vi "Forebrain.vi"() -> ()   [LabVIEW 2012]
uses:
  <vilib>/Utility/inputDevices.llb/closeKeyboard.vi
  <vilib>/Utility/inputDevices.llb/keyboardAcquire.vi
panel:
  in  "MANUAL \nOVERRIDE":bool
  out "Starboard Speed":i32(knob) scale=1000.0..2000.0
  out "Port Speed":i32(knob) scale=1000.0..2000.0
  in  "Rudders":i32(slide)=1500 scale=500.0..2500.0
  in  "Step Size":i32=5
  out "Speed                    Balance":i32(knob) scale=-1000.0..1000.0
  in  "Pan Camera":i32(slide)=1500 scale=500.0..2500.0
  in  "FULL STOP":bool
  out "UDP Timeout":bool
  out "UDP Working":bool
  in  "ESTOP":bool
  in  "PC Status":i32=1
  out "Port Rudder":i32
  out "Starboard Rudder":i32
  out "Port Motor":i32
  out "Starboard Motor":i32
  out "Data from XBEE":dbl
  out "XBEE Working":bool
  out "return count":u32
  out "Sent from XBEE":string
  out "bytes written":u32
  in  "Send to XBEE":string
  in  "VISA resource name":refnum<visa-resource-name>="COM6"
  in  "error in":errorcluster
  out "Base Station data rec'd":string
  out "Robot Stats":i32[](array[numeric])
  out "Buoy locations":cluster{"regular expression":string, i32, i32}[](array[cluster])
  # "ORGANIZE FRONT PANEL"
  # "Tug X"
  # "Tug Y"
  # "Tug H"
  # "MANUAL OVERRIDE CONTROLS"
  # "Controls:\nUse W/S to independently\ncontrol port speed.\nUse I/K to independently\ncontrol starboard speed.\nUse arrow keys to jointly\ncontrol motor speeds.\n\nUSE ESCAPE TO KILL MOTORS."
  # "Affects weight of single key input."
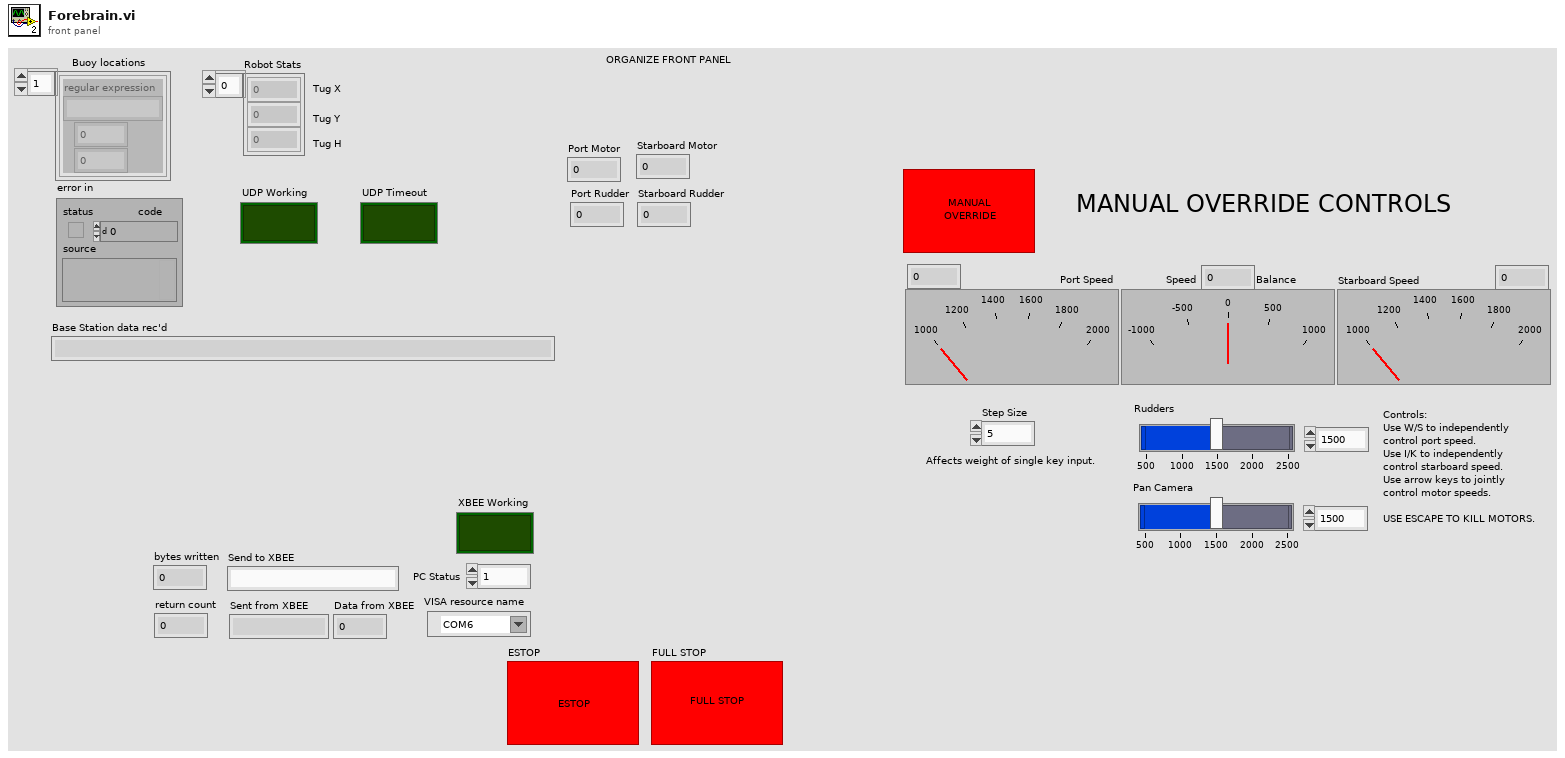
[diagram p1: front panel]
types:
  T1 = enum16{"0", "1", "2", "3", "4", "5", "6", "7", "8", "9", "A", "B", "C", "D", "E", "F", "G", "H", "I", "J", "K", "L", "M", "N", "O", "P", "Q", "R", "S", "T", "U", "V", "W", "X", "Y", "Z", "F1", "F2", "F3", "F4", "F5", "F6", "F7", "F8", "F9", "F10", "F11", "F12", "F13", "F14", "F15", "ADD", "BACK", "BACKSLASH", "CAPITAL", "COMMA", "DECIMAL", "DELETE", "DIVIDE", "DOWN", "END", "EQUALS", "ESCAPE", "GRAVE (`)", "HOME", "INSERT", "LBRACKET", "LCONTROL", "LEFT", "L ALT", "LSHIFT", "LWIN", "MINUS", "MULTIPLY", "NEXT", "NUMLOCK", "NUMPAD_0", "NUMPAD_1", "NUMPAD_2", "NUMPAD_3", "NUMPAD_4", "NUMPAD_5", "NUMPAD_6", "NUMPAD_7", "NUMPAD_8", "NUMPAD_9", "PAUSE", "PERIOD", "PRIOR (PG UP)", "RBRACKET", "RCONTROL", "RETURN", "RIGHT", "R ALT", "RSHIFT", "RWIN", "SCROLL", "SEMICOLON", "SLASH", "SPACE", "SUBTRACT", "TAB", "UP", "ENTER (num pad)", "' (quote)"}[]
  T2 = enum16{"0", "1", "2", "3", "4", "5", "6", "7", "8", "9", "A", "B", "C", "D", "E", "F", "G", "H", "I", "J", "K", "L", "M", "N", "O", "P", "Q", "R", "S", "T", "U", "V", "W", "X", "Y", "Z", "F1", "F2", "F3", "F4", "F5", "F6", "F7", "F8", "F9", "F10", "F11", "F12", "F13", "F14", "F15", "ADD", "BACK", "BACKSLASH", "CAPITAL", "COMMA", "DECIMAL", "DELETE", "DIVIDE", "DOWN", "END", "EQUALS", "ESCAPE", "GRAVE (`)", "HOME", "INSERT", "LBRACKET", "LCONTROL", "LEFT", "L ALT", "LSHIFT", "LWIN", "MINUS", "MULTIPLY", "NEXT", "NUMLOCK", "NUMPAD_0", "NUMPAD_1", "NUMPAD_2", "NUMPAD_3", "NUMPAD_4", "NUMPAD_5", "NUMPAD_6", "NUMPAD_7", "NUMPAD_8", "NUMPAD_9", "PAUSE", "PERIOD", "PRIOR (PG UP)", "RBRACKET", "RCONTROL", "RETURN", "RIGHT", "R ALT", "RSHIFT", "RWIN", "SCROLL", "SEMICOLON", "SLASH", "SPACE", "SUBTRACT", "TAB", "UP", "ENTER (num pad)", "' (quote)"}
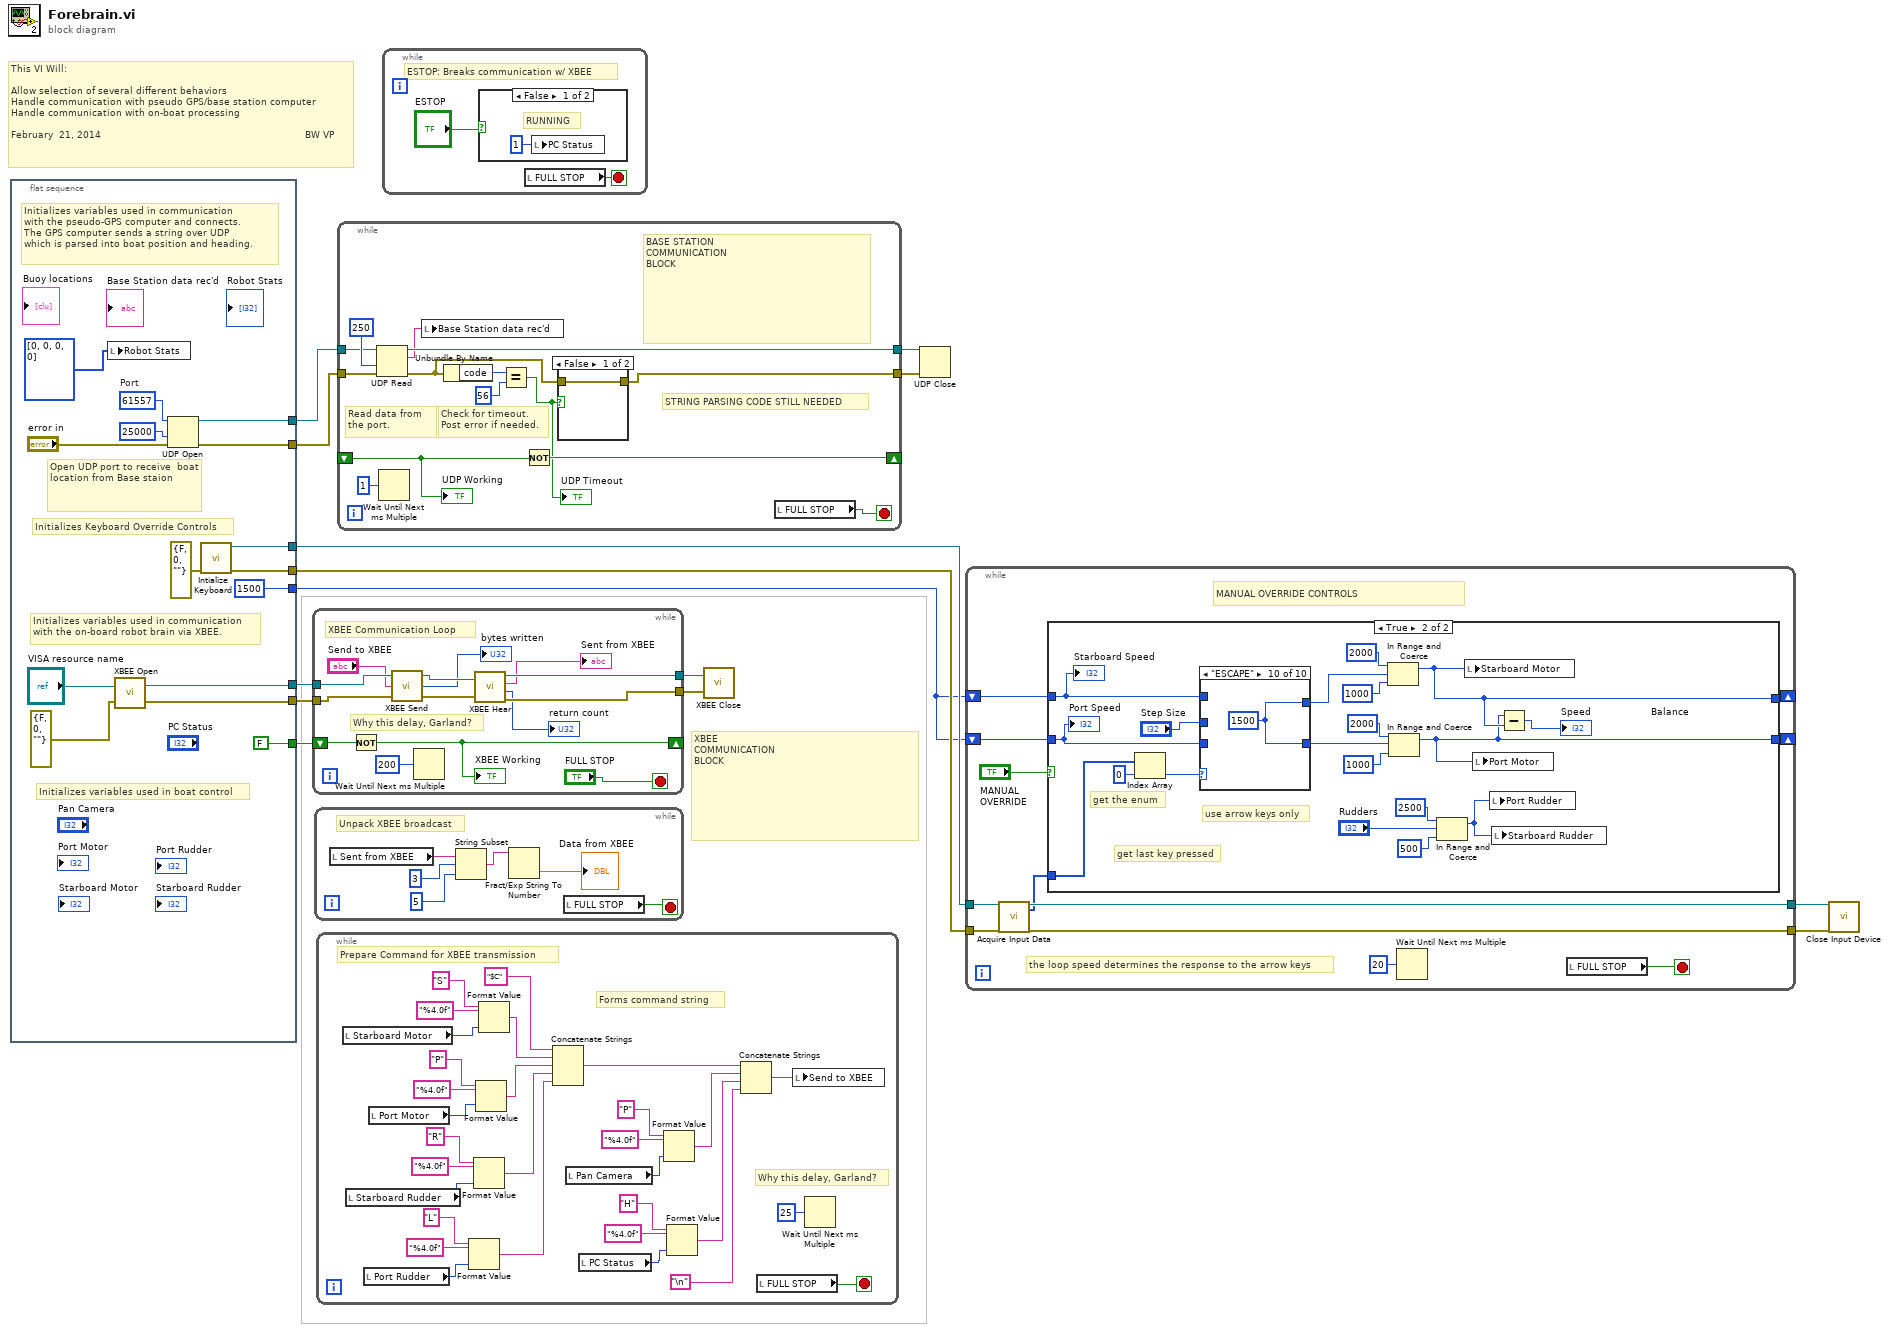
[diagram p0: block diagram]
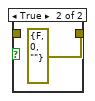
[diagram p2: hidden frame]
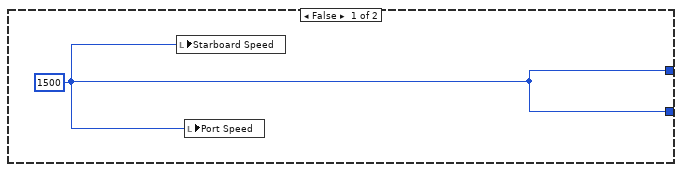
[diagram p3: hidden frame]
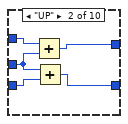
[diagram p5: hidden frame]
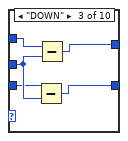
[diagram p6: hidden frame]
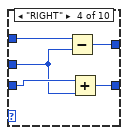
[diagram p7: hidden frame]
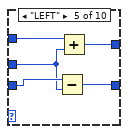
[diagram p8: hidden frame]
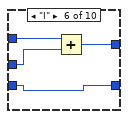
[diagram p9: hidden frame]
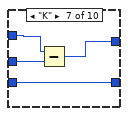
[diagram p10: hidden frame]
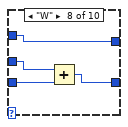
[diagram p11: hidden frame]
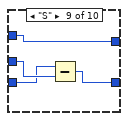
[diagram p12: hidden frame]
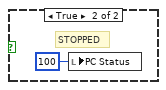
[diagram p13: hidden frame]
diagram:
  # "XBEE \nCOMMUNICATION\nBLOCK"
  # "This VI Will:\n\nAllow selection of several different behaviors\nHandle communication with pseudo GPS/base station computer\nHandle communication with on-boat processing\n\nFebruary  21, 2014                                                                    BW VP"
  n1 = flat-sequence {
    tunnel: [w25] -> w2
    tunnel: [w24] -> w1
    tunnel: [w21] -> w14
    tunnel: [w20] -> w13
    tunnel: [FALSE] -> w10
    tunnel: [w17] -> w7
    tunnel: [w16] -> w6
    tunnel: [1500] -> w5
    frame #0 {
      w28 = u16 61557  # Port
      # "Initializes Keyboard Override Controls"
      # "Initializes variables used in boat control"
      # "Initializes variables used in communication\nwith the on-board robot brain via XBEE."
      # "Initializes variables used in communication\nwith the pseudo-GPS computer and connects.\nThe GPS computer sends a string over UDP\nwhich is parsed into boat position and heading."
      # "Open UDP port to receive  boat location from Base staion"
      n2 = local write "Robot Stats"(i32[] [0, 0, 0, 0]) -> ()
      n3 = call "XBEE Open.vi"("error in"=errorcluster {"status"=FALSE, "code"=0, "source"=""}, "VISA resource name"="VISA resource name") -> ("error out"=w20:errorcluster, "VISA resource name out"=w21:refnum<visa-resource-name>)
      n4 = UDP Open(8:"error in", 9:25000 ("timeout ms (25000)"), 11:w28) -> (port=w25:refnum<k16>, 0:w24:errorcluster)  [unwired: 2 in, 1 out]
      n5 = call <vilib>:"Intialize Keyboard.vi"("error in (no error)"=errorcluster {"status"=FALSE, "code"=0, "source"=""}) -> ("error out"=w16:errorcluster, "device ID"=w17:refnum<k1>)  [unwired: 9 in]
    }
  }
  n6 = while {
    tunnel: w14 -> [w43]
    tunnel: w13 -> [w42]
    tunnel: [w37] -> w12
    tunnel: [w36] -> w11
    shift-right: [w31] -> _
    shift-left: w10 -> [w33]
    stop <- "FULL STOP" stop-if-true
    # "Why this delay, Garland?"
    # "XBEE Communication Loop"
    n7 = Not(x=w33) -> (.not. x?=w31:bool)
    "XBEE Working" <- w31
    n8 = call "XBEE Send.vi"("error in (no error)"=w42, "String"="Send to XBEE", "VISA resource name"=w43) -> ("error out"=w39:errorcluster, "return count"=→"bytes written":u32, "VISA resource name out"=w40:refnum<visa-resource-name>)
    n9 = Wait Until Next ms Multiple(millisecond multiple=200) -> ()  [unwired: 1 out]
    n10 = call "XBEE Hear.vi"("VISA resource name"=w40, "error in (no error)"=w39) -> ("VISA resource name out"=w37:refnum<visa-resource-name>, "String Received"=→"Sent from XBEE":string, "return count"=→"return count":u32, "error out"=w36:errorcluster)
  }
  n11 = while {
    stop <- w49 stop-if-true
    # "Unpack XBEE broadcast"
    n12 = local read "Sent from XBEE"() -> (w48:string)
    n13 = String Subset(string=w48, offset (0)=3, length (rest)=5 ("length (rest)")) -> (substring=w45:string)
    n14 = Fract/Exp String To Number(string=w45) -> (number=→"Data from XBEE":dbl)  [unwired: 3 in, 1 out]
    n15 = local read "FULL STOP"() -> (w49:bool)
  }
  n16 = while {
    stop <- w79 stop-if-true
    # "Why this delay, Garland?"
    # "Prepare Command for XBEE transmission"
    # "Forms command string"
    n17 = local read "Starboard Motor"() -> (w76:i32)
    n18 = local read "Starboard Rudder"() -> (w67:i32)
    n19 = local read "Port Rudder"() -> (w64:i32)
    n20 = local read "Port Motor"() -> (w73:i32)
    n21 = Format Value(string ("")="L", format string="%4.0f", value (0)=w64) -> (output string=w62:string)
    n22 = Format Value(string ("")="R", format string="%4.0f", value (0)=w67) -> (output string=w63:string)
    n23 = Format Value(string ("")="P", format string="%4.0f", value (0)=w73) -> (output string=w70:string)
    n24 = Format Value(string ("")="S", format string="%4.0f", value (0)=w76) -> (output string=w71:string)
    n25 = Concatenate Strings("$C", w71, w70, w63, w62) -> (w54:string)
    n26 = local read "Pan Camera"() -> (w58:i32)
    n27 = local read "PC Status"() -> (w55:i32)
    n28 = Format Value(string ("")="P", format string="%4.0f", value (0)=w58) -> (output string=w53:string)
    n29 = Format Value(string ("")="H", format string="%4.0f", value (0)=w55) -> (output string=w52:string)
    n30 = Concatenate Strings(w54, w53, w52, "\n") -> (w59:string)
    n31 = local read "FULL STOP"() -> (w79:bool)
    n32 = local write "Send to XBEE"(w59) -> ()
    n33 = Wait Until Next ms Multiple(millisecond multiple=u32 25) -> ()  [unwired: 1 out]
  }
  n34 = while {
    shift-right: [w91] -> _
    shift-left: _ -> [w81]
    tunnel: [w90] -> w4
    tunnel: [w86] -> w3
    tunnel: w2 -> [w84]
    tunnel: w1 -> [w83]
    stop <- w82 stop-if-true
    # "BASE STATION \nCOMMUNICATION\nBLOCK"
    # "Check for timeout.\nPost error if needed."
    # "Read data from\nthe port."
    # "STRING PARSING CODE STILL NEEDED"
    n35 = UDP Read(connection ID=w84, timeout ms (25000)=250, 8:w83) -> (data out=w85:string, error out=w87:errorcluster, 3:w90:refnum<k16>)  [unwired: 1 in, 2 out]
    n36 = Wait Until Next ms Multiple(millisecond multiple=u32 1) -> ()  [unwired: 1 out]
    n37 = local write "Base Station data rec'd"(w85) -> ()
    n38 = Unbundle By Name(w87) -> ("code"=w89:i32)
    n39 = Equal?(x=w89, y=56) -> (x = y?=w80:bool)
    "UDP Timeout" <- w80
    n40 = Not(x=w81) -> (.not. x?=w91:bool)
    n41 = case shown="False" w80 {
      tunnel: w87 -> [w94 _]
      tunnel: [w94 errorcluster {"status"=FALSE, "code"=0, "source"=""} ("error out")] -> w86
      frame False {
      }
      frame True {
      }
    }
    n42 = local read "FULL STOP"() -> (w82:bool)
    "UDP Working" <- w81
  }
  n43 = while {
    stop <- w97 stop-if-true
    # "ESTOP: Breaks communication w/ XBEE"
    n44 = case shown="False" "ESTOP" {
      frame False {
        # "RUNNING"
        n45 = local write "PC Status"(1 ("PC Status")) -> ()
      }
      frame True {
        # "STOPPED"
        n46 = local write "PC Status"(100) -> ()
      }
    }
    n47 = local read "FULL STOP"() -> (w97:bool)
  }
  n48 = call "XBEE Close.vi"("error in (no error)"=w11, "VISA resource name"=w12) -> ()
  n49 = UDP Close(connection ID=w4, 8:w3) -> ()  [unwired: 2 out]
  n50 = while {
    tunnel: [w111] -> w8
    tunnel: [w110] -> w9
    shift-right: [w104] -> _
    shift-left: w5 -> [w107]
    shift-right: [w103] -> _
    shift-left: w5 -> [w106]
    tunnel: w7 -> [w102]
    tunnel: w6 -> [w101]
    stop <- w105 stop-if-true
    # "MANUAL OVERRIDE CONTROLS"
    # "the loop speed determines the response to the arrow keys"
    n51 = call-poly <vilib>:"Acquire Input Data.vi"("device ID"=w102, "error in (no error)"=w101) -> ("device ID"=w110:refnum<k1>, "keys pressed"=w109:T1, "error out"=w111:errorcluster)  [unwired: 15 in]
    n52 = case shown="True" "MANUAL \nOVERRIDE" {
      tunnel: w109 -> [_ w131]
      tunnel: w107 -> [_ w128]
      tunnel: w106 -> [_ w127]
      tunnel: [w112 w115] -> w104
      tunnel: [w112 w114] -> w103
      frame False {
        w112 = 1500
        n53 = local write "Starboard Speed"(w112) -> ()
        n54 = local write "Port Speed"(w112) -> ()
      }
      frame True {
        # "use arrow keys only"
        # "get the enum"
        # "get last key pressed"
        n55 = Index Array(array=w131, index=0) -> (element=w129:T2)
        n56 = case shown="\"ESCAPE\"" w129 {
          tunnel: w128 -> [w133 w138 w143 w145 w150 w157 w159 w162 w166 _]
          tunnel: [w133 w137 w142 w146 w151 w156 w158 w162 w166 w170] -> w126
          tunnel: w127 -> [w132 w135 w140 w148 w152 w154 w161 w164 w168 _]
          tunnel: [w132 w134 w139 w147 w153 w154 w161 w163 w167 w170] -> w117
          tunnel: "Step Size" -> [_ w136 w141 w144 w149 w155 w160 w165 w169 _]
          frame "0", Default {
          }
          frame "UP" {
            n57 = Add(x=w138, y=w136) -> (x+y=w137:i32)
            n58 = Add(x=w136, y=w135) -> (x+y=w134:i32)
          }
          frame "DOWN" {
            n59 = Subtract(x=w140, y=w141) -> (x-y=w139:i32)
            n60 = Subtract(x=w143, y=w141) -> (x-y=w142:i32)
          }
          frame "RIGHT" {
            n61 = Subtract(x=w145, y=w144) -> (x-y=w146:i32)
            n62 = Add(x=w148, y=w144) -> (x+y=w147:i32)
          }
          frame "LEFT" {
            n63 = Subtract(x=w152, y=w149) -> (x-y=w153:i32)
            n64 = Add(x=w150, y=w149) -> (x+y=w151:i32)
          }
          frame "I" {
            n65 = Add(x=w157, y=w155) -> (x+y=w156:i32)
          }
          frame "K" {
            n66 = Subtract(x=w159, y=w160) -> (x-y=w158:i32)
          }
          frame "W" {
            n67 = Add(x=w165, y=w164) -> (x+y=w163:i32)
          }
          frame "S" {
            n68 = Subtract(x=w168, y=w169) -> (x-y=w167:i32)
          }
          frame "ESCAPE" {
            w170 = 1500
          }
        }
        n69 = In Range and Coerce(upper limit=2000, x=w126, lower limit=1000) -> (coerced(x)=w115:i32)  [unwired: 1 out]
        n70 = In Range and Coerce(upper limit=2000, x=w117, lower limit=1000) -> (coerced(x)=w114:i32)  [unwired: 1 out]
        n71 = In Range and Coerce(upper limit=2500, x="Rudders", lower limit=500) -> (coerced(x)=w113:i32)  [unwired: 1 out]
        n72 = local write "Starboard Motor"(w115) -> ()
        n73 = local write "Port Motor"(w114) -> ()
        n74 = local write "Port Rudder"(w113) -> ()
        n75 = local write "Starboard Rudder"(w113) -> ()
        n76 = Subtract(x=w114, y=w115) -> (x-y=→"Speed                    Balance":i32)
        "Starboard Speed" <- w128
        "Port Speed" <- w127
      }
    }
    n77 = Wait Until Next ms Multiple(millisecond multiple=u32 20) -> ()  [unwired: 1 out]
    n78 = local read "FULL STOP"() -> (w105:bool)
  }
  n79 = call-poly <vilib>:"Close Input Device.vi"("error in (no error)"=w8, "device ID"=w9) -> ()  [unwired: 8 in, 1 out]
